vi "Send Frame.vi"(8 "entrée d'erreur (pas d'erreur)":errorcluster, 11 "Send_Frame en entrée":refnum<class "Zigbee_Send_Command_UART.lvclass">) -> (0 "sortie d'erreur":errorcluster, 3 "Send_Frame en sortie":refnum<class "Zigbee_Send_Command_UART.lvclass">)   [LabVIEW 2020, in "Library Test.lvlib" / "Zigbee_Send_Command_UART.lvclass"]
uses:
  Zigbee_Send_Command_UART.lvclass
  C:/Users/ngarcin/OneDrive - Altyor/Standard TB/Suite TB45/Class/Test/Test (Default)/Test (Default).lvclass
  Commun VI/TypeDef/Variable Printable.ctl
  JSON API/Variant JSON/Variant to JSON.vi
  JSON API/JSON Value/Get Item by name array.vi
  Instrument/Instrument (Default)/Class Instrument (Default).lvclass
  JSON API/JSON Value/JSON Value.lvclass
  JSON API/Get Polymorphic/JSON GetSet.lvlib
  Commun VI/Library Commun.lvlib
  JSON API/Variant JSON/Variant JSON.lvlib
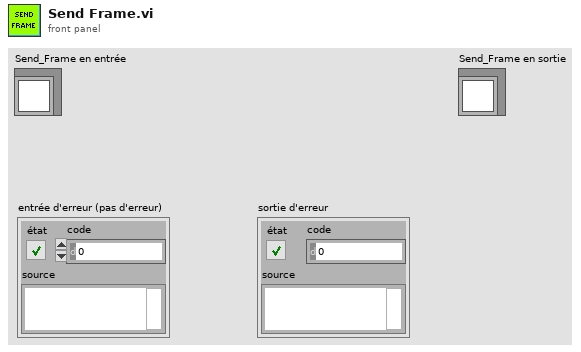
[diagram p1: front panel]
types:
  T1 = typedef "Variable Printable.ctl" = string
  T2 = enum16{"Get Variable", "Get All Variables", "Set Variable", "Delete Variable", "Delete All Variable"}
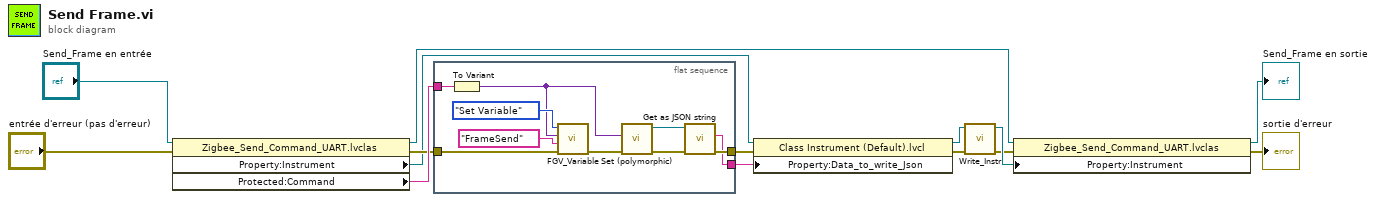
[diagram p0: block diagram]
diagram:
  n1 = property class="Zigbee_Send_Command_UART.lvclas"(reference="Send_Frame en entrée", error in="entrée d'erreur (pas d'erreur)") -> (reference out=w4:refnum<class "Zigbee_Send_Command_UART.lvclass">, error out=w7:errorcluster, "Property:Instrument"=w2:refnum<class "Class Instrument (Default).lvclass">, "Protected:Command"=w9:string)
  n2 = flat-sequence {
    tunnel: [w24] -> w13
    tunnel: [w23] -> w12
    tunnel: w9 -> [w16]
    tunnel: w7 -> [w17]
    frame #0 {
      n3 = To Variant(anything=w16) -> (Variant=w15:variant)
      n4 = call "FGV_Variable.vi"("error in (no error)"=w17, "Variable"=T1 "FrameSend", "Data In"=w15, "Function"=T2."Set Variable") -> ("error out"=w18:errorcluster)  [unwired: 5 in, 2 out]
      n5 = call-poly "Set (polymorphic).vi"("error in (no error)"=w18, "Variant"=w15) -> ("error out"=w22:errorcluster, "JSON Value out"=w21:refnum<class "JSON Value.lvclass">)  [unwired: 8 in]
      n6 = call "Get as JSON string.vi"("error in (no error)"=w22, "JSON Value in"=w21) -> ("error out"=w24:errorcluster, "<JSON>"=w23:string)  [unwired: 8 in]
    }
  }
  n7 = property class="Class Instrument (Default).lvcl"(reference=w2, error in=w13, "Property:Data_to_write_Json"=w12) -> (reference out=w11:refnum<class "Class Instrument (Default).lvclass">, error out=w14:errorcluster)
  n8 = call-dynamic "Write_Instr.vi"("error in (no error)"=w14, "Class Multimeter (Default) en entrée"=w11) -> ("error out"=w1:errorcluster, "Class Multimeter (Default) en sortie"=w5:refnum<class "Class Instrument (Default).lvclass">)  [unwired: 8 in]
  n9 = property class="Zigbee_Send_Command_UART.lvclas"(reference=w4, error in=w1, "Property:Instrument"=w5) -> (reference out=→"Send_Frame en sortie":refnum<class "Zigbee_Send_Command_UART.lvclass">, error out=→"sortie d'erreur":errorcluster)
